vi "Temperature Logger.vi"() -> ()   [LabVIEW 2018]
uses:
  <vilib>/Analysis/baseanly.llb/Mean (DBL).vi
  <vilib>/Analysis/NI_AALBase.lvlib
panel:
  in  "stop":bool
  out "Current Index":dbl
  out "Mean Temp":dbl
  out "Min Temp":dbl
  out "Max Temp":dbl
  out "Current Data":dbl(slide) scale=0.0..100.0
  in  "Temp Scale":bool
  # "Deg C"
  # "Deg F"
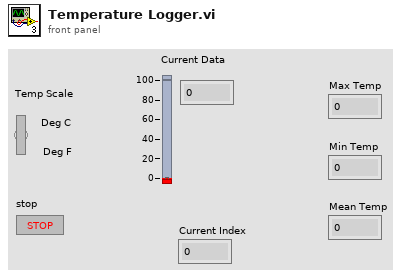
[diagram p1: front panel]
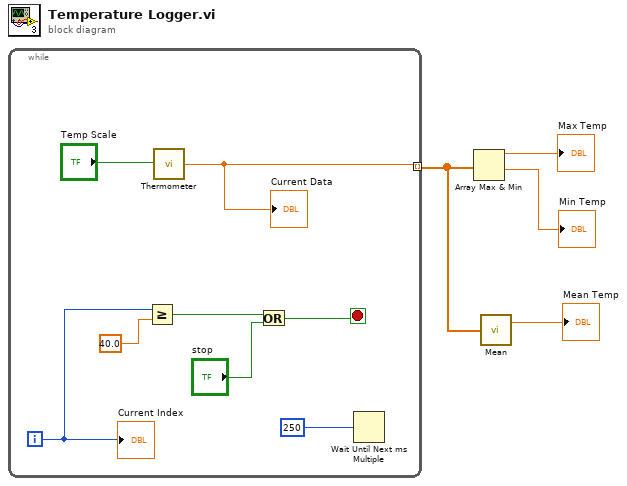
[diagram p0: block diagram]
diagram:
  n1 = while {
    tunnel: [w5] -> w2 mode=indexing
    i -> [w10]
    stop <- w7 stop-if-true
    n2 = Greater Or Equal?(x=w10, y=40.0) -> (x >= y?=w9:bool)
    n3 = call "Thermometer.vi"("Temp Scale"="Temp Scale") -> ("Temperature"=w5:dbl)
    "Current Data" <- w5
    n4 = Or(x=w9, y="stop") -> (x .or. y?=w7:bool)
    n5 = Wait Until Next ms Multiple(millisecond multiple=250) -> ()  [unwired: 1 out]
    "Current Index" <- w10
  }
  n6 = Array Max & Min(array=w2) -> (max value=→"Max Temp":dbl, min value=→"Min Temp":dbl)  [unwired: 2 out]
  n7 = call-poly <vilib>:"Mean.vi"("X"=w2) -> ("mean"=→"Mean Temp":dbl)  [unwired: 1 out]
